vi "IsServerRunning.vi"(8 "error in (no error)":errorcluster, 11 "Server in":refnum<class "Server.lvclass">) -> (0 "error out":errorcluster, 2 "RunTime":u64, 3 "Server out":refnum<class "Server.lvclass">)   [LabVIEW 2017, in "opcua.lvlib" / "Server.lvclass"]
uses:
  Server.lvclass
  Server.lvclass/Server.ctl
  opcua32.dll
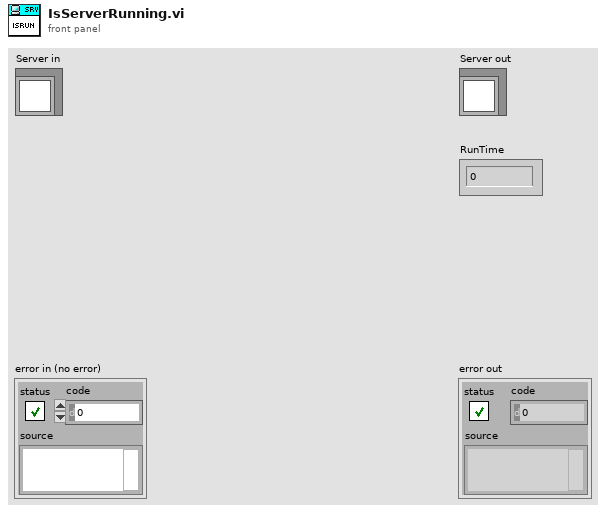
[diagram p1: front panel]
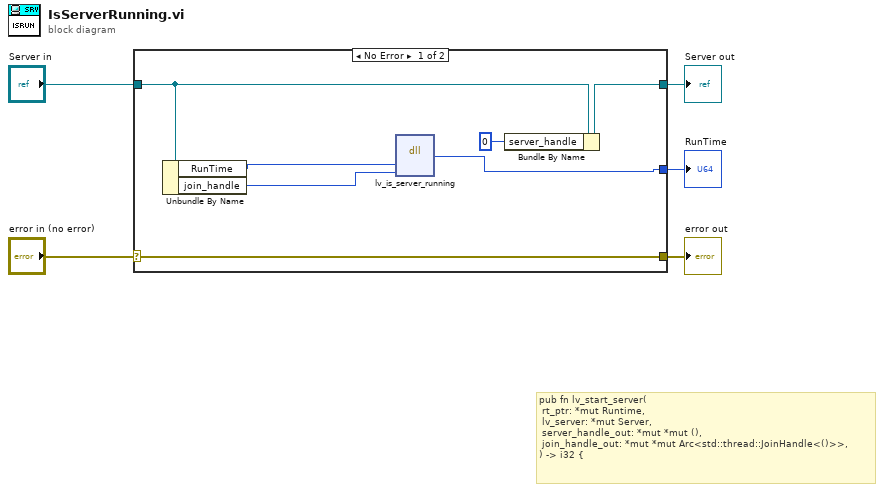
[diagram p0: block diagram]
diagram:
  # "pub fn lv_start_server(\n\trt_ptr: *mut Runtime,\n\tlv_server: *mut Server,\n\tserver_handle_out: *mut *mut (),\n\tjoin_handle_out: *mut *mut Arc<std::thread::JoinHandle<()>>,\n) -> i32 {"
  n1 = case shown="No Error" "error in (no error)" {
    selector: "error in (no error)" -> [w12 w13]
    tunnel: [w12 w13] -> w4
    tunnel: [w8 w14] -> w2
    tunnel: "Server in" -> [w9 w14]
    tunnel: [w7 _] -> w1
    frame No Error {
      n2 = Unbundle By Name(w9) -> ("RunTime"=w11:u64, "join_handle"=w10:u64)
      n3 = dll-call lib="C:/Users/Andrey/Desktop/opcua-labview/opcua-lvlib/opcua*.dll" fn="lv_is_server_running"("RunTime"=w11, "handle_join"=w10) -> ("return type"=w7:i32)  [unwired: 5 in, 2 out]
      n4 = Bundle By Name(cluster=w9, "server_handle"=u64 0) -> (w8:refnum<class "Server.lvclass">)
    }
    frame Error {
    }
  }
  "error out" <- w4
  "Server out" <- w2
  "RunTime" <- w1
